vi "CRYHardware Mic Start.vi"(0 "Setup in":T6={"No.VI"=0, "Category"="", "StepName"="", "Seq setup flattened"="", "Comment"="", "Steps config."=[], "Jump config"=[], "Start"=0.0, "Increment"=0.0, "Name"="Pa", "Unit"="Pa", "Y data"=1, "Y prefix"="", "Y dB ref"=1.0, "Y unit"="", "Repeat State Array"=[]} {"Repeat State Array"."Start" format="%#_5g"; "Y dB ref" format="%.1f"; "Y data" items=["dB", "Lin"]; "Start" format="%#_5g"}, 5 "Data in":T4 {"Z data" items=["dB", "Lin"]; "X data" items=["dB", "Lin"]; "Y data" items=["dB", "Lin"]; "Z dB ref" format="%.1f"; "Z axis" items=["Log", "Lin"]; "X dB ref" format="%.1f"; "X axis" items=["Log", "Lin"]; "Y axis" items=["Log", "Lin"]; "Y dB ref" format="%.1f"; "Curve"."z" format="%.2f"; "Curve"."y" format="%.2f"; "Curve"."x" format="%.2f"}, 7 "Results in":T2 {"Margin" format="%.2f"}, 9 "Seq Setup in":string, 11 "Step name":string, 12 "Hardware in":string, 13 "Calibration in":string) -> (3 "Types Out":string[](array[string]), 4 "Inserted Names Out":string[](array[string]), 6 "Data out":T4 {"Z data" items=["dB", "Lin"]; "X data" items=["dB", "Lin"]; "Y data" items=["dB", "Lin"]; "Z dB ref" format="%.1f"; "Z axis" items=["Log", "Lin"]; "X dB ref" format="%.1f"; "X axis" items=["Log", "Lin"]; "Y axis" items=["Log", "Lin"]; "Y dB ref" format="%.1f"; "Curve"."z" format="%.2f"; "Curve"."y" format="%.2f"; "Curve"."x" format="%.2f"}, 8 "Results out":T2 {"Margin" format="%.2f"}, 10 "Wave out":T1[](array[typedef]) {"Y dB ref" format="%.1f"; "Y axis" items=["Log", "Lin"]; "Y data" items=["dB", "Lin"]; "X data" items=["dB", "Lin"]})   [LabVIEW 2013]
uses:
  Typedef Control/CRYData Cluster Array.ctl
  Typedef Control/CRYData Cluster.ctl
  Typedef Control/CRYResult Cluster Array.ctl
  Typedef Control/CRYResult Cluster.ctl
  Typedef Control/CRYStep.ctl
  Typedef Control/CRYWaveform Cluster.ctl
  CRYHardware Global.vi
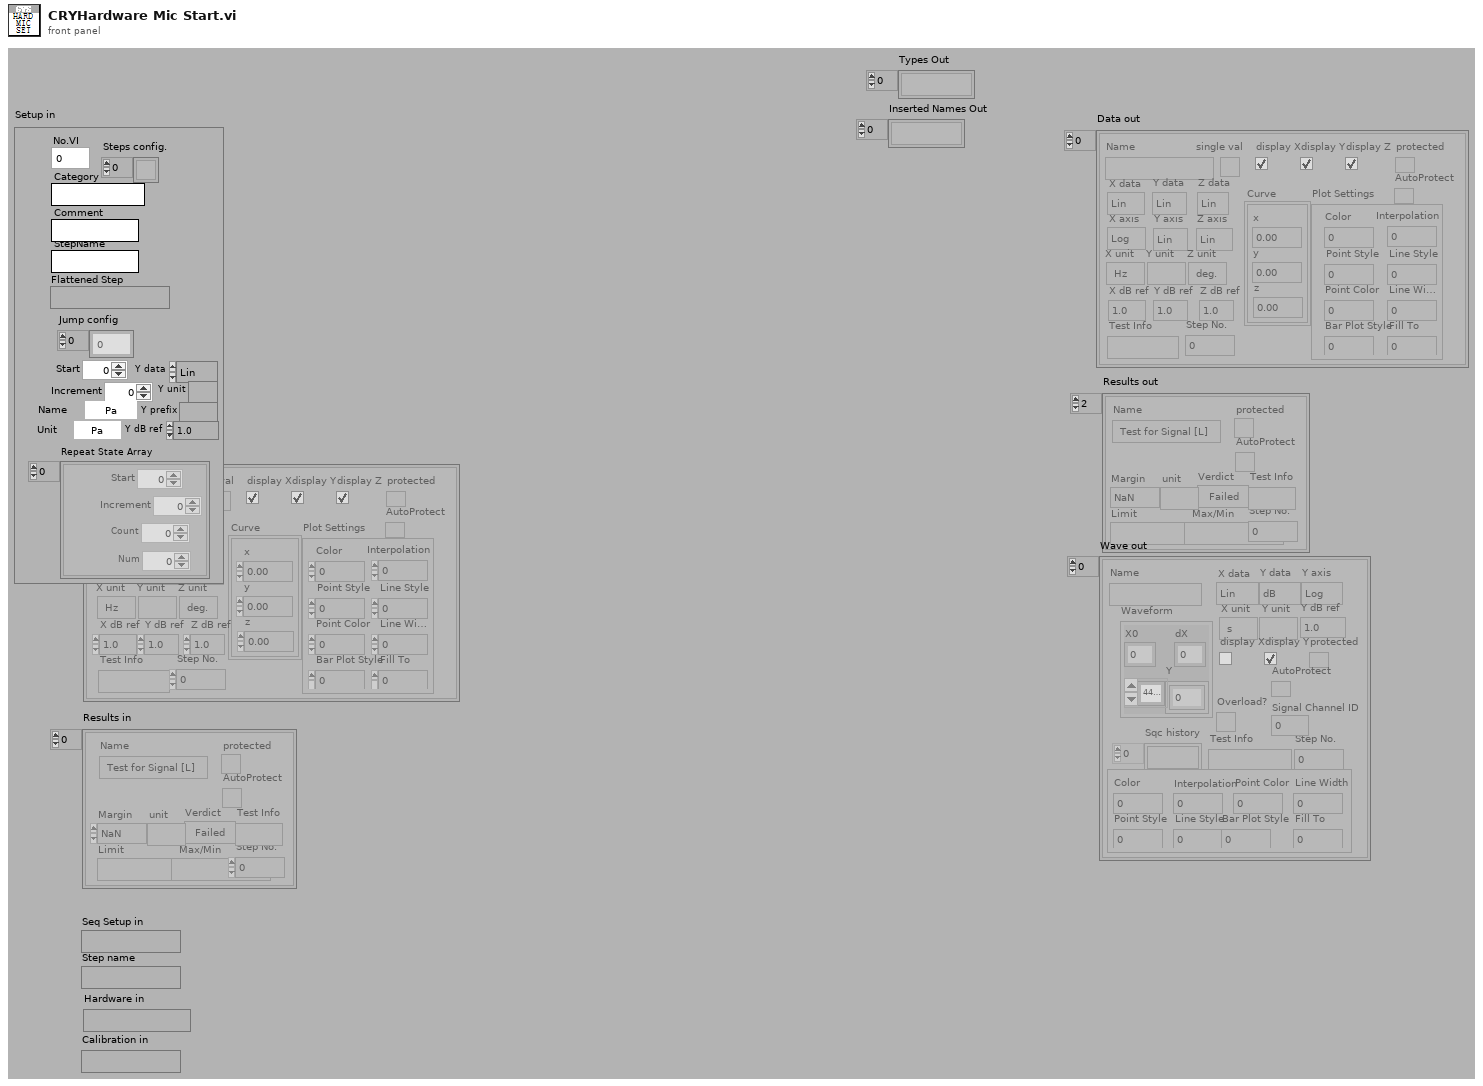
[diagram p1: front panel]
types:
  T1 = typedef "CRYWaveform Cluster.ctl" = cluster{"Waveform":cluster{"X0":dbl, "dX":dbl, "Y":sgl[]}, "X data":u16, "Y data":u16, "Y axis":u16, "X unit":string, "Y unit":string, "Y dB ref":dbl, "display Y":bool, "display X":bool, "Overload?":bool, "Test Info":string, "Step No.":i32, "Name":string, "protected":bool, "Sqc history":string[], "Signal Channel ID":i32, "Plot Settings":cluster{"Color":u32, "Interpolation":u8, "Point Style":u8, "Line Style":u8, "Point Color":u32, "Line Width":u8, "Bar Plot Style":u8, "Fill To":i16}, "AutoProtect":bool}
  T2 = typedef "CRYResult Cluster Array.ctl" = T3[]
  T3 = typedef "CRYResult Cluster.ctl" = cluster{"Name":string, "Margin":dbl, "unit":string, "Verdict":bool, "Limit":string, "Max/Min":string, "protected":bool, "Step No.":i32, "Test Info":string, "AutoProtect":bool}
  T4 = typedef "CRYData Cluster Array.ctl" = T5[]
  T5 = typedef "CRYData Cluster.ctl" = cluster{"Name":string, "Curve":cluster{"x":dbl, "y":dbl, "z":dbl}[], "X data":u16, "Y data":u16, "Z data":u16, "X axis":u16, "Y axis":u16, "Z axis":u16, "X unit":string, "Y unit":string, "Z unit":string, "X dB ref":dbl, "Y dB ref":dbl, "Z dB ref":dbl, "single val":bool, "protected":bool, "display X":bool, "display Y":bool, "display Z":bool, "Test Info":string, "Step No.":i32, "Plot Settings":cluster{"Color":u32, "Interpolation":u8, "Point Style":u8, "Line Style":u8, "Point Color":u32, "Line Width":u8, "Bar Plot Style":u8, "Fill To":i16}, "AutoProtect":bool}
  T6 = typedef "CRYStep.ctl" = cluster{"No.VI":i32, "Category":string, "StepName":string, "Seq setup flattened":string, "Comment":string, "Steps config.":bool[], "Jump config":i32[], "Start":dbl, "Increment":dbl, "Name":string, "Unit":string, "Y data":u16, "Y prefix":string, "Y dB ref":dbl, "Y unit":string, "Repeat State Array":cluster{"Start":dbl, "Increment":dbl, "Count":i32, "Num":i32}[]}
  T7 = typedef "CRY6175Hardware.ctl" = cluster{"Tab Value":u16, "Help":string, "In Channel 1":u16, "In Channel 2":u16, "In Gain 1":i32, "In Gain 2":i32, "Mic Volt":i32, "Mic Resis":i32, "Out Channel":u16, "OUT_Impedance 1":u16, "OUT_Impedance 2":u16, "IN_Channel 1 Old":u16}
  T8 = enum16{"OK", "Yes", "YesNo", "YesNoCancel", "ReplaceAppend"}
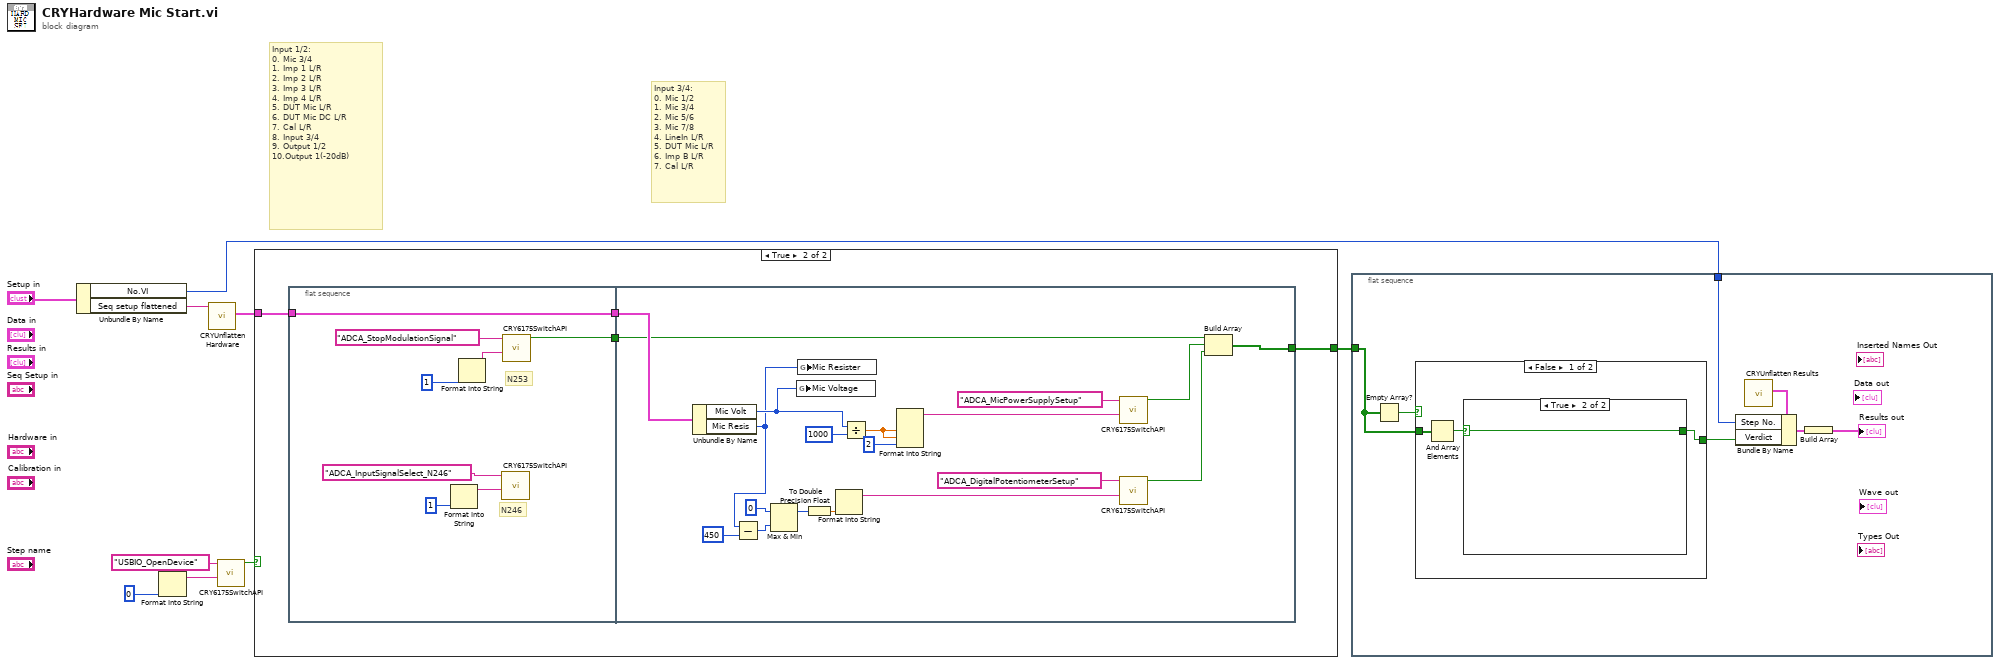
[diagram p0: block diagram]
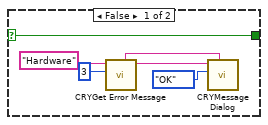
[diagram p2: hidden frame]
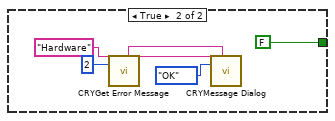
[diagram p3: hidden frame]
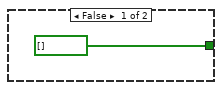
[diagram p4: hidden frame]
diagram:
  # "Input 3/4:\n0. Mic 1/2\n1. Mic 3/4\n2. Mic 5/6\n3. Mic 7/8\n4. LineIn L/R\n5. DUT Mic L/R\n6. Imp B L/R\n7. Cal L/R"
  # "Input 1/2:\n0. Mic 3/4\n1. Imp 1 L/R\n2. Imp 2 L/R\n3. Imp 3 L/R\n4. Imp 4 L/R\n5. DUT Mic L/R\n6. DUT Mic DC L/R\n7. Cal L/R\n8. Input 3/4\n9. Output 1/2 \n10.Output 1(-20dB)"
  n1 = Unbundle By Name("Setup in") -> ("No.VI"=w2:i32, "Seq setup flattened"=w8:string)
  n2 = Format Into String(0) -> (resulting string=w3:string)  [unwired: 3 in, 1 out]
  n3 = call "CRYUnflatten Hardware.vi"("Unflatten Hardware#"=w8) -> ("Hardware"=w6:T7)  [unwired: 8 in, 2 out]
  n4 = call "CRY6175SwitchAPI.vi"("Parameter"=w3, "Function Name"="USBIO_OpenDevice") -> ("bResult"=w1:bool)  [unwired: 9 in]
  n5 = case shown="True" w1 {
    tunnel: w6 -> [_ w13]
    tunnel: [bool[] [] w14] -> w7
    frame False {
    }
    frame True {
      n6 = flat-sequence {
        tunnel: w13 -> [w22]
        tunnel: [w22] -> w12
        tunnel: [w18] -> w11
        tunnel: [w30] -> w14
        tunnel: w12 -> [w33]
        tunnel: w11 -> [w29]
        frame #0 {
          # "N246"
          # "N253"
          n7 = Format Into String(u16 1 ("In Channel 1")) -> (resulting string=w15:string)  [unwired: 3 in, 1 out]
          n8 = Format Into String(u16 1 ("input 1")) -> (resulting string=w20:string)  [unwired: 3 in, 1 out]
          n9 = call "CRY6175SwitchAPI.vi"("Parameter"=w15, "Function Name"="ADCA_InputSignalSelect_N246") -> ()  [unwired: 9 in, 1 out]
          n10 = call "CRY6175SwitchAPI.vi"("Parameter"=w20, "Function Name"="ADCA_StopModulationSignal") -> ("bResult"=w18:bool)  [unwired: 9 in]
        }
        frame #1 {
          n11 = Unbundle By Name(w33) -> ("Mic Volt"=w24:i32, "Mic Resis"=w23:i32)
          n12 = Subtract(x=w23, y=450) -> (x-y=w27:i32)
          n13 = Max & Min(x=0 ("y"), y=w27) -> (max(x,y)=w25:i32)  [unwired: 1 out]
          n14 = global write "CRYHardware Global.vi" "Mic Voltage"(w24) -> ()
          n15 = global write "CRYHardware Global.vi" "Mic Resister"(w23) -> ()
          n16 = To Double Precision Float(number=w25) -> (double precision float=w40:dbl)
          n17 = Format Into String(w40) -> (resulting string=w41:string)  [unwired: 3 in, 1 out]
          n18 = Divide(x=w24, y=1000) -> (x/y=w37:dbl)
          n19 = Format Into String(w37, w37, 2 ("input 3")) -> (resulting string=w39:string)  [unwired: 3 in, 1 out]
          n20 = call "CRY6175SwitchAPI.vi"("Parameter"=w39, "Function Name"="ADCA_MicPowerSupplySetup") -> ("bResult"=w32:bool)  [unwired: 9 in]
          n21 = call "CRY6175SwitchAPI.vi"("Parameter"=w41, "Function Name"="ADCA_DigitalPotentiometerSetup") -> ("bResult"=w31:bool)  [unwired: 9 in]
          n22 = Build Array(w29, w32, w31) -> (w30:bool[])
        }
      }
    }
  }
  n23 = flat-sequence {
    tunnel: w7 -> [w44]
    tunnel: w2 -> [w42]
    frame #0 {
      n24 = Empty Array?(array=w44) -> (empty?=w46:bool)
      n25 = case shown="False" w46 {
        tunnel: w44 -> [w51 _]
        tunnel: [w49 FALSE ("empty?")] -> w45
        frame False {
          n26 = And Array Elements(Boolean array=w51) -> (logical AND=w50:bool)
          n27 = case shown="True" w50 {
            selector: w50 -> [w52 w58]
            tunnel: [w52 w58] -> w49
            frame False {
              n28 = call "CRYGet Error Message.vi"("Error No"=3, "Kind"="Hardware") -> ("Message"=w54:string, "Window Title"=w55:string)  [unwired: 4 in, 4 out]
              n29 = call "CRYMessage Dialog.vi"("Window Title"=w55, "YesNoCancel"=T8."OK", "Message Content"=w54) -> ()  [unwired: 7 in, 2 out]
            }
            frame True {
            }
          }
        }
        frame True {
          n30 = call "CRYGet Error Message.vi"("Error No"=2, "Kind"="Hardware") -> ("Message"=w61:string, "Window Title"=w62:string)  [unwired: 4 in, 4 out]
          n31 = call "CRYMessage Dialog.vi"("Window Title"=w62, "YesNoCancel"=T8."OK", "Message Content"=w61) -> ()  [unwired: 7 in, 2 out]
        }
      }
      n32 = call "CRYUnflatten Results.vi"() -> ("Result"=w48:T3)  [unwired: 9 in, 2 out]
      n33 = Bundle By Name(cluster=w48, "Step No."=w42, "Verdict"=w45) -> (w47:T3)
      n34 = Build Array(w47) -> (→"Results out":T3[])
    }
  }
